vi "FS Body.vi"   [LabVIEW 2019]
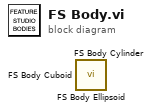
[diagram p0: block diagram]
diagram:
  n1 = call <userlib>:"FS Body Ellipsoid.vi"() -> ()  [unwired: 11 in, 1 out]
  n2 = call <userlib>:"FS Body Cylinder.vi"() -> ()  [unwired: 11 in, 1 out]
  n3 = call <userlib>:"FS Body Cuboid.vi"() -> ()  [unwired: 11 in, 1 out]
